vi "CreateXmlFromReadings.vi"(8 "error in":errorcluster) -> (0 "error out":errorcluster, 3 "xml string":string)   [LabVIEW 2016]
uses:
  processVariables.ctl
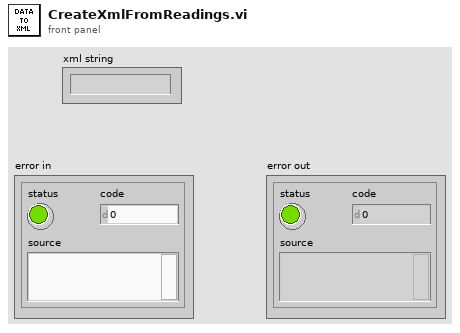
[diagram p1: front panel]
types:
  T1 = typedef "processVariables.ctl" = cluster{"Level":dbl, "Aeration":bool, "Feed":bool, "Mixer":bool, "Overflow":bool, "Recycle":bool, "Substrate":bool, "CO2_3000ppm":dbl, "Mixing":dbl, "pH":dbl, "Temperature":dbl, "Redox":dbl, "Turbidity":dbl, "Oxygen":dbl, "Flow":dbl, "CO2_10000ppm":dbl, "Aeration_percentage":dbl}
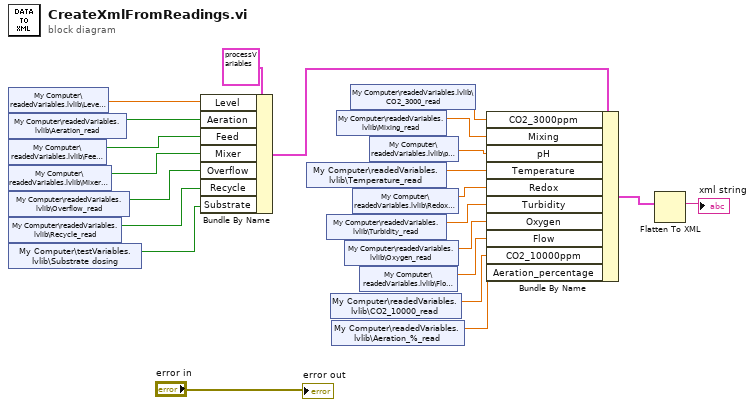
[diagram p0: block diagram]
diagram:
  n1 = shared-variable "My Computer\\readedVariables.lvlib\\Level_read"() -> (w21:dbl)  [unwired: 1 in, 1 out]
  n2 = shared-variable "My Computer\\readedVariables.lvlib\\Aeration_read"() -> (w18:bool)  [unwired: 1 in, 1 out]
  n3 = shared-variable "My Computer\\readedVariables.lvlib\\Feed_read"() -> (w17:bool)  [unwired: 1 in, 1 out]
  n4 = shared-variable "My Computer\\readedVariables.lvlib\\Mixer_read"() -> (w16:bool)  [unwired: 1 in, 1 out]
  n5 = shared-variable "My Computer\\readedVariables.lvlib\\Overflow_read"() -> (w15:bool)  [unwired: 1 in, 1 out]
  n6 = shared-variable "My Computer\\readedVariables.lvlib\\Recycle_read"() -> (w14:bool)  [unwired: 1 in, 1 out]
  n7 = shared-variable "My Computer\\testVariables.lvlib\\Substrate dosing"() -> (w13:bool)  [unwired: 1 in, 1 out]
  n8 = Bundle By Name(cluster=T1 {"Level"=0.0, "Aeration"=FALSE, "Feed"=FALSE, "Mixer"=FALSE, "Overflow"=FALSE, "Recycle"=FALSE, "Substrate"=FALSE, "CO2_3000ppm"=0.0, "Mixing"=0.0, "pH"=0.0, "Temperature"=0.0, "Redox"=0.0, "Turbidity"=0.0, "Oxygen"=0.0, "Flow"=0.0, "CO2_10000ppm"=0.0, "Aeration_percentage"=0.0} ("Cluster"), "Level"=w21, "Aeration"=w18, "Feed"=w17, "Mixer"=w16, "Overflow"=w15, "Recycle"=w14, "Substrate"=w13) -> (w12:T1)
  n9 = shared-variable "My Computer\\readedVariables.lvlib\\Temperature_read"() -> (w7:dbl)  [unwired: 1 in, 1 out]
  n10 = shared-variable "My Computer\\readedVariables.lvlib\\Turbidity_read"() -> (w5:dbl)  [unwired: 1 in, 1 out]
  n11 = shared-variable "My Computer\\readedVariables.lvlib\\CO2_10000_read"() -> (w2:dbl)  [unwired: 1 in, 1 out]
  n12 = shared-variable "My Computer\\readedVariables.lvlib\\Aeration_%_read"() -> (w1:dbl)  [unwired: 1 in, 1 out]
  n13 = shared-variable "My Computer\\readedVariables.lvlib\\Mixing_read"() -> (w9:dbl)  [unwired: 1 in, 1 out]
  n14 = shared-variable "My Computer\\readedVariables.lvlib\\Oxygen_read"() -> (w11:dbl)  [unwired: 1 in, 1 out]
  n15 = shared-variable "My Computer\\readedVariables.lvlib\\CO2_3000_read"() -> (w10:dbl)  [unwired: 1 in, 1 out]
  n16 = shared-variable "My Computer\\readedVariables.lvlib\\Redox_read"() -> (w6:dbl)  [unwired: 1 in, 1 out]
  n17 = shared-variable "My Computer\\readedVariables.lvlib\\Flow_read"() -> (w3:dbl)  [unwired: 1 in, 1 out]
  n18 = shared-variable "My Computer\\readedVariables.lvlib\\pH_read"() -> (w8:dbl)  [unwired: 1 in, 1 out]
  n19 = Bundle By Name(cluster=w12, "CO2_3000ppm"=w10, "Mixing"=w9, "pH"=w8, "Temperature"=w7, "Redox"=w6, "Turbidity"=w5, "Oxygen"=w11, "Flow"=w3, "CO2_10000ppm"=w2, "Aeration_percentage"=w1) -> (w4:T1)
  n20 = Flatten To XML(anything=w4) -> (xml string=→"xml string":string)
  "error out" <- "error in"
